vi "test-linear-system-id.vi"() -> ()   [LabVIEW 2019]
uses:
  <vilib>/Rock Robotics/WPI/ThirdParty/JAS_Junk/TrajLib/LINEAR_SYSTEM.ctl
  <vilib>/Analysis/Matrix/Datatypes/RealMatrix.ctl
  <vilib>/Rock Robotics/WPI/ThirdParty/JAS_Junk/TrajLib/MatBuilder_Create.vi
  <vilib>/Rock Robotics/WPI/ThirdParty/JAS_Junk/TrajLib/MatrixHelper_Zero.vi
  <vilib>/Rock Robotics/WPI/ThirdParty/JAS_Junk/TrajLib/DCMotor_New.vi
  <vilib>/Rock Robotics/WPI/ThirdParty/JAS_Junk/TrajLib/Units_RotationsPerMinuteToRadiansPerSecond.vi
  <vilib>/Rock Robotics/WPI/ThirdParty/JAS_Junk/TrajLib/Matrix_Ident.vi
  <vilib>/Rock Robotics/WPI/ThirdParty/JAS_Junk/TrajLib/LinearSystem_New.vi
  <vilib>/Analysis/7linalg.llb/Create Special Matrix.vi
  <vilib>/Analysis/7linalg.llb/Create Special Real Matrix.vi
  <vilib>/Rock Robotics/WPI/ThirdParty/JAS_Junk/TrajLib/Trajectory_Library.lvlib
  <vilib>/Analysis/Matrix/NI_Matrix.lvlib
panel:
  out "T D 5":bool
  out "T C 5":bool
  out "T B 5":bool
  out "T A 5":bool
  out "T D 4":bool
  out "T C 4":bool
  out "T B 4":bool
  out "T A 4":bool
  out "T D 3":bool
  out "T C 3":bool
  out "T B 3":bool
  out "T A 3":bool
  out "T D 2":bool
  out "T C 2":bool
  out "T B 2":bool
  out "T A 2":bool
  out "T D 1":bool
  out "T C 1":bool
  out "T B 1":bool
  out "T A 1":bool
  out "IdentifyVelocitySystem":T1
  out "IdentifyPositionSystem":T1
  out "FlyWheel":T1
  out "DriveTrain":T1
  out "Elevator":T1
  # "A  = -10.14132, 3.06598, \n            3.06598, -10.14132\n\nB =    4.2590,   -1.28762, \n         -1.2876,   4.2590\n\nC =   1.0,   0.0, \n          0.0,  1.0;\n\nD =   0.0,   0.0, \n          0.0,   0.0"
  # "A   = (0, 1, \n               0, -99.05473)\n\n     B = (0, \n            20.8)\n\n   C   = 1, 0\n\n    D = 0"
  # "A = -26.87032\n\nB = 1354.166667;\n\nC = 1\n\nD = 0"
  # "A =   0, 1, \n         0, -1 / 0.5\n\nB =  0, \n        1 / 0.5"
  # "A =   -1.0 / 0.5\n\nB = 1 / 0.5"
  # "<States,States>"
  # "<States,Inputs>"
  # "<Outputs,States>"
  # "<Outputs,Inputs>"
  # "<States,States>"
  # "<States,Inputs>"
  # "<Outputs,States>"
  # "<Outputs,Inputs>"
  # "<States,States>"
  # "<States,Inputs>"
  # "<Outputs,States>"
  # "<Outputs,Inputs>"
  # "<States,States>"
  # "<States,Inputs>"
  # "<Outputs,States>"
  # "<Outputs,Inputs>"
  # "<States,States>"
  # "<States,Inputs>"
  # "<Outputs,States>"
  # "<Outputs,Inputs>"
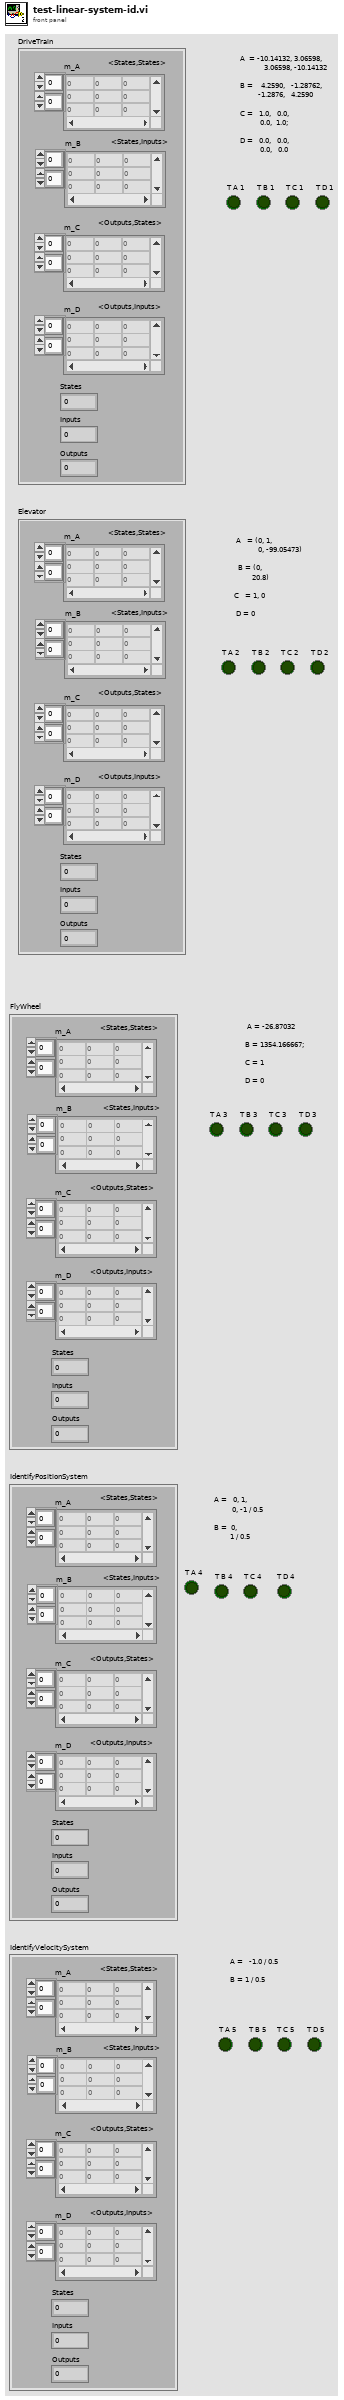
[diagram p1: front panel]
types:
  T1 = typedef "Trajectory_Library.lvlib/LINEAR_SYSTEM.ctl" = cluster{"m_A":T2, "m_B":T2, "m_C":T2, "m_D":T2, "States":i32, "Inputs":i32, "Outputs":i32}
  T2 = typedef "NI_Matrix.lvlib/RealMatrix.ctl" = dbl[][]
  T3 = typedef "Trajectory_Library.lvlib/DCMOTOR.CTL" = cluster{"nominalVoltage_Volts":dbl, "StallTorque_NM":dbl, "StallCurrent_Amps":dbl, "FreeCurrent_Amps":dbl, "FreeSpeed_RadPerSec":dbl, "R_Ohms":dbl, "Kv_RadPerSecPerVolt":dbl, "Kt_NMPerAmp":dbl}
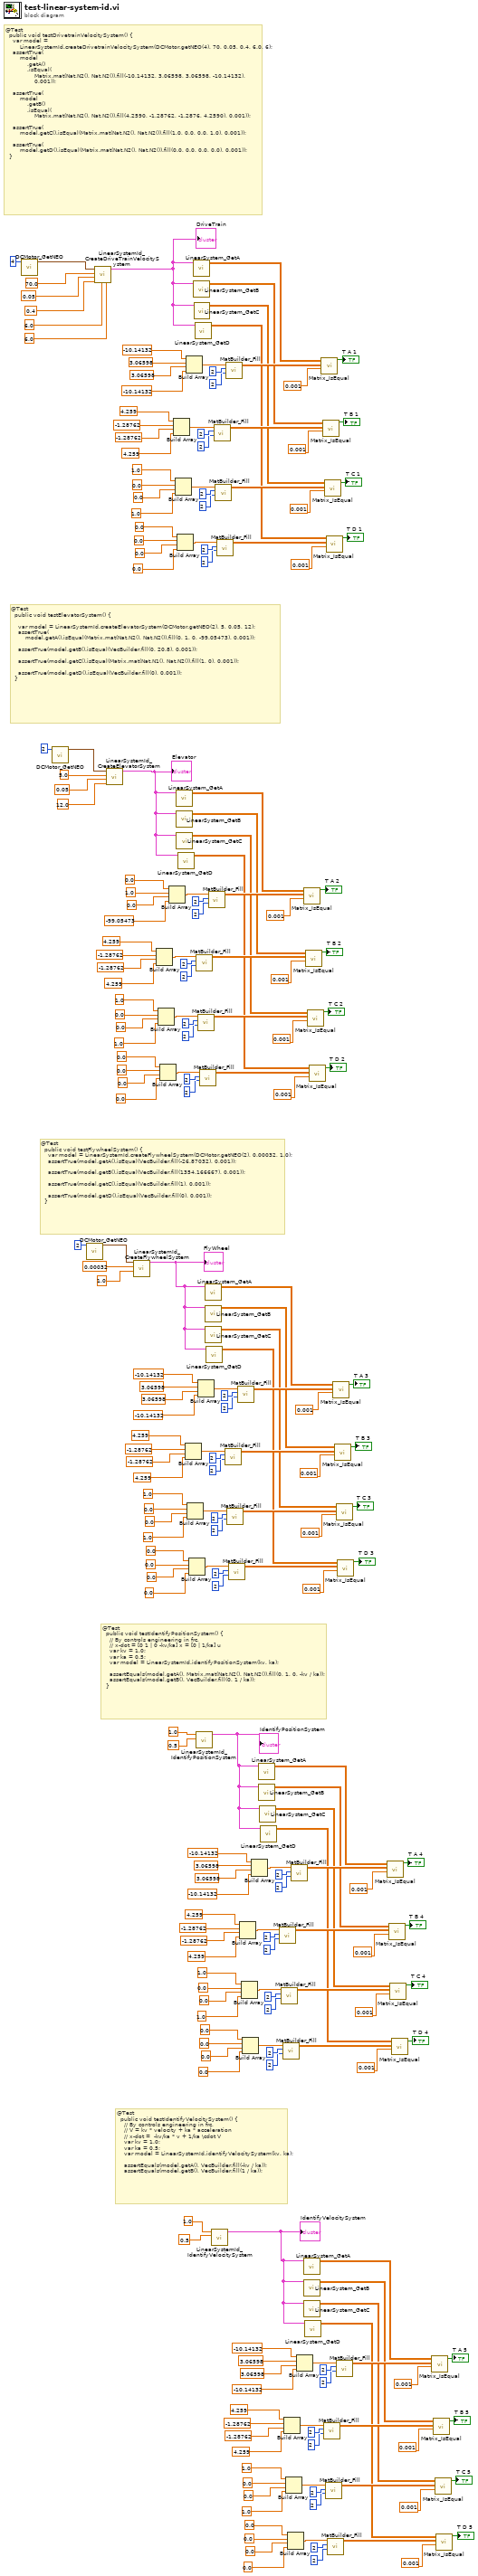
[diagram p0: block diagram]
diagram:
  # "@Test\n  public void testIdentifyVelocitySystem() {\n    // By controls engineering in frc,\n    // V = kv * velocity + ka * acceleration\n    // x-dot =  -kv/ka * v + 1/ka \\cdot V\n    var kv = 1.0;\n    var ka = 0.5;\n    var model = LinearSystemId.identifyVelocitySystem(kv, ka);\n\n    assertEquals(model.getA(), VecBuilder.fill(-kv / ka));\n    assertEquals(model.getB(), VecBuilder.fill(1 / ka));"
  # "@Test\n  public void testIdentifyPositionSystem() {\n    // By controls engineering in frc,\n    // x-dot = [0 1 | 0 -kv/ka] x = [0 | 1/ka] u\n    var kv = 1.0;\n    var ka = 0.5;\n    var model = LinearSystemId.identifyPositionSystem(kv, ka);\n\n    assertEquals(model.getA(), Matrix.mat(Nat.N2(), Nat.N2()).fill(0, 1, 0, -kv / ka));\n    assertEquals(model.getB(), VecBuilder.fill(0, 1 / ka));\n  }"
  # "@Test\n  public void testFlywheelSystem() {\n    var model = LinearSystemId.createFlywheelSystem(DCMotor.getNEO(2), 0.00032, 1.0);\n    assertTrue(model.getA().isEqual(VecBuilder.fill(-26.87032), 0.001));\n\n    assertTrue(model.getB().isEqual(VecBuilder.fill(1354.166667), 0.001));\n\n    assertTrue(model.getC().isEqual(VecBuilder.fill(1), 0.001));\n\n    assertTrue(model.getD().isEqual(VecBuilder.fill(0), 0.001));\n  }"
  # "@Test\n  public void testDrivetrainVelocitySystem() {\n    var model =\n        LinearSystemId.createDrivetrainVelocitySystem(DCMotor.getNEO(4), 70, 0.05, 0.4, 6.0, 6);\n    assertTrue(\n        model\n            .getA()\n            .isEqual(\n                Matrix.mat(Nat.N2(), Nat.N2()).fill(-10.14132, 3.06598, 3.06598, -10.14132),\n                0.001));\n\n    assertTrue(\n        model\n            .getB()\n            .isEqual(\n                Matrix.mat(Nat.N2(), Nat.N2()).fill(4.2590, -1.28762, -1.2876, 4.2590), 0.001));\n\n    assertTrue(\n        model.getC().isEqual(Matrix.mat(Nat.N2(), Nat.N2()).fill(1.0, 0.0, 0.0, 1.0), 0.001));\n\n    assertTrue(\n        model.getD().isEqual(Matrix.mat(Nat.N2(), Nat.N2()).fill(0.0, 0.0, 0.0, 0.0), 0.001));\n  }"
  # "@Test\n  public void testElevatorSystem() {\n\n    var model = LinearSystemId.createElevatorSystem(DCMotor.getNEO(2), 5, 0.05, 12);\n    assertTrue(\n        model.getA().isEqual(Matrix.mat(Nat.N2(), Nat.N2()).fill(0, 1, 0, -99.05473), 0.001));\n\n    assertTrue(model.getB().isEqual(VecBuilder.fill(0, 20.8), 0.001));\n\n    assertTrue(model.getC().isEqual(Matrix.mat(Nat.N1(), Nat.N2()).fill(1, 0), 0.001));\n\n    assertTrue(model.getD().isEqual(VecBuilder.fill(0), 0.001));\n  }"
  n1 = call <vilib>:"DCMotor_GetNEO.vi"("Num Motors"=4) -> ("DCMOTOR"=w239:T3)  [unwired: 10 in]
  n2 = call <vilib>:"DCMotor_GetNEO.vi"("Num Motors"=2) -> ("DCMOTOR"=w244:T3)  [unwired: 10 in]
  n3 = call <vilib>:"DCMotor_GetNEO.vi"("Num Motors"=2) -> ("DCMOTOR"=w232:T3)  [unwired: 10 in]
  n4 = call <vilib>:"LinearSystemId_CreateDriveTrainVelocitySystem.vi"("G"=6.0, "JKgMetersSquared"=6.0, "rbMeters"=0.4, "rMeters"=0.05, "MassKg"=70.0, "Motor"=w239) -> ("Linearsystem"=w203:T1)  [unwired: 4 in, 1 out]
  "DriveTrain" <- w203
  n5 = call <vilib>:"LinearSystemId_CreateElevatorSystem.vi"("G"=12.0, "radiusMeters"=0.05, "massKg"=5.0, "DCMOTOR"=w244) -> ("Linearsystem"=w136:T1)  [unwired: 6 in, 1 out]
  "Elevator" <- w136
  n6 = call <vilib>:"LinearSystemId_CreateFlywheelSystem.vi"("G"=1.0, "jKgMetersSquared"=0.00032, "DCMOTOR"=w232) -> ("Linearsystem"=w91:T1)  [unwired: 7 in, 1 out]
  "FlyWheel" <- w91
  n7 = Build Array(4.259 ("element"), -1.28762 ("element"), -1.28762 ("element"), 4.259 ("element")) -> (w169:dbl[])
  n8 = Build Array(1.0 ("element"), 0.0 ("element"), 0.0 ("element"), 1.0 ("element")) -> (w158:dbl[])
  n9 = Build Array(0.0 ("element"), 0.0 ("element"), 0.0 ("element"), 0.0 ("element")) -> (w148:dbl[])
  n10 = Build Array(0.0 ("element"), 1.0 ("element"), 0.0 ("element"), -99.05473 ("element")) -> (w180:dbl[])
  n11 = Build Array(4.259 ("element"), -1.28762 ("element"), -1.28762 ("element"), 4.259 ("element")) -> (w214:dbl[])
  n12 = Build Array(1.0 ("element"), 0.0 ("element"), 0.0 ("element"), 1.0 ("element")) -> (w202:dbl[])
  n13 = call <vilib>:"LinearSystem_GetA.vi"("Linearsystem"=w136) -> ("A"=w173:T2)  [unwired: 10 in]
  n14 = call <vilib>:"LinearSystem_GetB.vi"("Linearsystem"=w136) -> ("B"=w159:T2)  [unwired: 10 in]
  n15 = call <vilib>:"LinearSystem_GetC.vi"("Linearsystem"=w136) -> ("C"=w138:T2)  [unwired: 10 in]
  n16 = Build Array(0.0 ("element"), 0.0 ("element"), 0.0 ("element"), 0.0 ("element")) -> (w192:dbl[])
  n17 = call <vilib>:"LinearSystem_GetD.vi"("Linearsystem"=w136) -> ("D"=w137:T2)  [unwired: 10 in]
  n18 = Build Array(4.259 ("element"), -1.28762 ("element"), -1.28762 ("element"), 4.259 ("element")) -> (w124:dbl[])
  n19 = Build Array(-10.14132 ("element"), 3.06598 ("element"), 3.06598 ("element"), -10.14132 ("element")) -> (w225:dbl[])
  n20 = Build Array(1.0 ("element"), 0.0 ("element"), 0.0 ("element"), 1.0 ("element")) -> (w113:dbl[])
  n21 = Build Array(0.0 ("element"), 0.0 ("element"), 0.0 ("element"), 0.0 ("element")) -> (w103:dbl[])
  n22 = call <vilib>:"LinearSystem_GetA.vi"("Linearsystem"=w203) -> ("A"=w218:T2)  [unwired: 10 in]
  n23 = call <vilib>:"LinearSystem_GetB.vi"("Linearsystem"=w203) -> ("B"=w204:T2)  [unwired: 10 in]
  n24 = call <vilib>:"LinearSystem_GetC.vi"("Linearsystem"=w203) -> ("C"=w182:T2)  [unwired: 10 in]
  n25 = call <vilib>:"LinearSystem_GetD.vi"("Linearsystem"=w203) -> ("D"=w181:T2)  [unwired: 10 in]
  n26 = call <vilib>:"LinearSystemId_IdentifyPositionSystem.vi"("kA"=0.5, "kV"=1.0) -> ("Linearsystem"=w46:T1)  [unwired: 8 in, 1 out]
  "IdentifyPositionSystem" <- w46
  n27 = call <vilib>:"MatBuilder_Fill.vi"("Columns"=2, "Rows"=2, "Value List"=w169) -> ("output matrix"=w162:T2)  [unwired: 6 in, 2 out]
  n28 = Build Array(-10.14132 ("element"), 3.06598 ("element"), 3.06598 ("element"), -10.14132 ("element")) -> (w135:dbl[])
  n29 = call <vilib>:"MatBuilder_Fill.vi"("Columns"=2, "Rows"=2, "Value List"=w158) -> ("output matrix"=w151:T2)  [unwired: 6 in, 2 out]
  n30 = call <vilib>:"MatBuilder_Fill.vi"("Columns"=2, "Rows"=2, "Value List"=w148) -> ("output matrix"=w141:T2)  [unwired: 6 in, 2 out]
  n31 = call <vilib>:"LinearSystem_GetA.vi"("Linearsystem"=w91) -> ("A"=w128:T2)  [unwired: 10 in]
  n32 = call <vilib>:"LinearSystem_GetB.vi"("Linearsystem"=w91) -> ("B"=w114:T2)  [unwired: 10 in]
  n33 = call <vilib>:"LinearSystem_GetC.vi"("Linearsystem"=w91) -> ("C"=w93:T2)  [unwired: 10 in]
  n34 = call <vilib>:"LinearSystem_GetD.vi"("Linearsystem"=w91) -> ("D"=w92:T2)  [unwired: 10 in]
  n35 = call <vilib>:"MatBuilder_Fill.vi"("Columns"=2, "Rows"=2, "Value List"=w180) -> ("output matrix"=w172:T2)  [unwired: 6 in, 2 out]
  n36 = call <vilib>:"LinearSystemId_IdentifyVelocitySystem.vi"("kA"=0.5, "kV"=1.0) -> ("Linearsystem"=w1:T1)  [unwired: 8 in, 1 out]
  "IdentifyVelocitySystem" <- w1
  n37 = call <vilib>:"MatBuilder_Fill.vi"("Columns"=2, "Rows"=2, "Value List"=w214) -> ("output matrix"=w207:T2)  [unwired: 6 in, 2 out]
  n38 = call <vilib>:"MatBuilder_Fill.vi"("Columns"=2, "Rows"=2, "Value List"=w202) -> ("output matrix"=w195:T2)  [unwired: 6 in, 2 out]
  n39 = call <vilib>:"MatBuilder_Fill.vi"("Columns"=2, "Rows"=2, "Value List"=w192) -> ("output matrix"=w185:T2)  [unwired: 6 in, 2 out]
  n40 = call <vilib>:"MatBuilder_Fill.vi"("Columns"=2, "Rows"=2, "Value List"=w124) -> ("output matrix"=w117:T2)  [unwired: 6 in, 2 out]
  n41 = call <vilib>:"MatBuilder_Fill.vi"("Columns"=2, "Rows"=2, "Value List"=w225) -> ("output matrix"=w217:T2)  [unwired: 6 in, 2 out]
  n42 = call <vilib>:"MatBuilder_Fill.vi"("Columns"=2, "Rows"=2, "Value List"=w113) -> ("output matrix"=w106:T2)  [unwired: 6 in, 2 out]
  n43 = call <vilib>:"MatBuilder_Fill.vi"("Columns"=2, "Rows"=2, "Value List"=w103) -> ("output matrix"=w96:T2)  [unwired: 6 in, 2 out]
  n44 = call <vilib>:"MatBuilder_Fill.vi"("Columns"=2, "Rows"=2, "Value List"=w135) -> ("output matrix"=w127:T2)  [unwired: 6 in, 2 out]
  n45 = Build Array(4.259 ("element"), -1.28762 ("element"), -1.28762 ("element"), 4.259 ("element")) -> (w79:dbl[])
  n46 = Build Array(1.0 ("element"), 0.0 ("element"), 0.0 ("element"), 1.0 ("element")) -> (w68:dbl[])
  n47 = Build Array(0.0 ("element"), 0.0 ("element"), 0.0 ("element"), 0.0 ("element")) -> (w58:dbl[])
  n48 = Build Array(-10.14132 ("element"), 3.06598 ("element"), 3.06598 ("element"), -10.14132 ("element")) -> (w90:dbl[])
  n49 = call <vilib>:"LinearSystem_GetA.vi"("Linearsystem"=w46) -> ("A"=w83:T2)  [unwired: 10 in]
  n50 = call <vilib>:"LinearSystem_GetB.vi"("Linearsystem"=w46) -> ("B"=w69:T2)  [unwired: 10 in]
  n51 = call <vilib>:"LinearSystem_GetC.vi"("Linearsystem"=w46) -> ("C"=w48:T2)  [unwired: 10 in]
  n52 = call <vilib>:"LinearSystem_GetD.vi"("Linearsystem"=w46) -> ("D"=w47:T2)  [unwired: 10 in]
  n53 = call <vilib>:"MatBuilder_Fill.vi"("Columns"=2, "Rows"=2, "Value List"=w79) -> ("output matrix"=w72:T2)  [unwired: 6 in, 2 out]
  n54 = call <vilib>:"MatBuilder_Fill.vi"("Columns"=2, "Rows"=2, "Value List"=w68) -> ("output matrix"=w61:T2)  [unwired: 6 in, 2 out]
  n55 = call <vilib>:"MatBuilder_Fill.vi"("Columns"=2, "Rows"=2, "Value List"=w58) -> ("output matrix"=w51:T2)  [unwired: 6 in, 2 out]
  n56 = Build Array(4.259 ("element"), -1.28762 ("element"), -1.28762 ("element"), 4.259 ("element")) -> (w34:dbl[])
  n57 = Build Array(1.0 ("element"), 0.0 ("element"), 0.0 ("element"), 1.0 ("element")) -> (w23:dbl[])
  n58 = Build Array(0.0 ("element"), 0.0 ("element"), 0.0 ("element"), 0.0 ("element")) -> (w13:dbl[])
  n59 = call <vilib>:"MatBuilder_Fill.vi"("Columns"=2, "Rows"=2, "Value List"=w90) -> ("output matrix"=w82:T2)  [unwired: 6 in, 2 out]
  n60 = Build Array(-10.14132 ("element"), 3.06598 ("element"), 3.06598 ("element"), -10.14132 ("element")) -> (w45:dbl[])
  n61 = call <vilib>:"LinearSystem_GetA.vi"("Linearsystem"=w1) -> ("A"=w38:T2)  [unwired: 10 in]
  n62 = call <vilib>:"LinearSystem_GetB.vi"("Linearsystem"=w1) -> ("B"=w24:T2)  [unwired: 10 in]
  n63 = call <vilib>:"Matrix_IsEqual.vi"("Tolerance"=0.001, "other"=w172, "input matrix"=w173) -> ("Equal"=→"T A 2":bool)  [unwired: 8 in]
  n64 = call <vilib>:"LinearSystem_GetC.vi"("Linearsystem"=w1) -> ("C"=w3:T2)  [unwired: 10 in]
  n65 = call <vilib>:"LinearSystem_GetD.vi"("Linearsystem"=w1) -> ("D"=w2:T2)  [unwired: 10 in]
  n66 = call <vilib>:"Matrix_IsEqual.vi"("Tolerance"=0.001, "other"=w162, "input matrix"=w159) -> ("Equal"=→"T B 2":bool)  [unwired: 8 in]
  n67 = call <vilib>:"Matrix_IsEqual.vi"("Tolerance"=0.001, "other"=w151, "input matrix"=w138) -> ("Equal"=→"T C 2":bool)  [unwired: 8 in]
  n68 = call <vilib>:"Matrix_IsEqual.vi"("Tolerance"=0.001, "other"=w141, "input matrix"=w137) -> ("Equal"=→"T D 2":bool)  [unwired: 8 in]
  n69 = call <vilib>:"Matrix_IsEqual.vi"("Tolerance"=0.001, "other"=w217, "input matrix"=w218) -> ("Equal"=→"T A 1":bool)  [unwired: 8 in]
  n70 = call <vilib>:"Matrix_IsEqual.vi"("Tolerance"=0.001, "other"=w207, "input matrix"=w204) -> ("Equal"=→"T B 1":bool)  [unwired: 8 in]
  n71 = call <vilib>:"MatBuilder_Fill.vi"("Columns"=2, "Rows"=2, "Value List"=w34) -> ("output matrix"=w27:T2)  [unwired: 6 in, 2 out]
  n72 = call <vilib>:"Matrix_IsEqual.vi"("Tolerance"=0.001, "other"=w195, "input matrix"=w182) -> ("Equal"=→"T C 1":bool)  [unwired: 8 in]
  n73 = call <vilib>:"MatBuilder_Fill.vi"("Columns"=2, "Rows"=2, "Value List"=w23) -> ("output matrix"=w16:T2)  [unwired: 6 in, 2 out]
  n74 = call <vilib>:"Matrix_IsEqual.vi"("Tolerance"=0.001, "other"=w185, "input matrix"=w181) -> ("Equal"=→"T D 1":bool)  [unwired: 8 in]
  n75 = call <vilib>:"MatBuilder_Fill.vi"("Columns"=2, "Rows"=2, "Value List"=w13) -> ("output matrix"=w6:T2)  [unwired: 6 in, 2 out]
  n76 = call <vilib>:"Matrix_IsEqual.vi"("Tolerance"=0.001, "other"=w127, "input matrix"=w128) -> ("Equal"=→"T A 3":bool)  [unwired: 8 in]
  n77 = call <vilib>:"Matrix_IsEqual.vi"("Tolerance"=0.001, "other"=w117, "input matrix"=w114) -> ("Equal"=→"T B 3":bool)  [unwired: 8 in]
  n78 = call <vilib>:"Matrix_IsEqual.vi"("Tolerance"=0.001, "other"=w106, "input matrix"=w93) -> ("Equal"=→"T C 3":bool)  [unwired: 8 in]
  n79 = call <vilib>:"MatBuilder_Fill.vi"("Columns"=2, "Rows"=2, "Value List"=w45) -> ("output matrix"=w37:T2)  [unwired: 6 in, 2 out]
  n80 = call <vilib>:"Matrix_IsEqual.vi"("Tolerance"=0.001, "other"=w96, "input matrix"=w92) -> ("Equal"=→"T D 3":bool)  [unwired: 8 in]
  n81 = call <vilib>:"Matrix_IsEqual.vi"("Tolerance"=0.001, "other"=w82, "input matrix"=w83) -> ("Equal"=→"T A 4":bool)  [unwired: 8 in]
  n82 = call <vilib>:"Matrix_IsEqual.vi"("Tolerance"=0.001, "other"=w72, "input matrix"=w69) -> ("Equal"=→"T B 4":bool)  [unwired: 8 in]
  n83 = call <vilib>:"Matrix_IsEqual.vi"("Tolerance"=0.001, "other"=w61, "input matrix"=w48) -> ("Equal"=→"T C 4":bool)  [unwired: 8 in]
  n84 = call <vilib>:"Matrix_IsEqual.vi"("Tolerance"=0.001, "other"=w51, "input matrix"=w47) -> ("Equal"=→"T D 4":bool)  [unwired: 8 in]
  n85 = call <vilib>:"Matrix_IsEqual.vi"("Tolerance"=0.001, "other"=w37, "input matrix"=w38) -> ("Equal"=→"T A 5":bool)  [unwired: 8 in]
  n86 = call <vilib>:"Matrix_IsEqual.vi"("Tolerance"=0.001, "other"=w27, "input matrix"=w24) -> ("Equal"=→"T B 5":bool)  [unwired: 8 in]
  n87 = call <vilib>:"Matrix_IsEqual.vi"("Tolerance"=0.001, "other"=w16, "input matrix"=w3) -> ("Equal"=→"T C 5":bool)  [unwired: 8 in]
  n88 = call <vilib>:"Matrix_IsEqual.vi"("Tolerance"=0.001, "other"=w6, "input matrix"=w2) -> ("Equal"=→"T D 5":bool)  [unwired: 8 in]
